vi "SVFA Power in Band.vi"   [LabVIEW 2017]
doc: "Computes the aggregate power in the <B>range</B>. The SVFA Power in Band VI operates on Power, PSD, COP, and FFT [Mag] spectra. Wire data to the <B>spectrum</B> input to determine the polymorphic instance to use or manually select the instance."
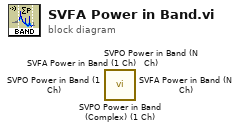
[diagram p0: block diagram]
diagram:
  n1 = call <vilib>:"SVPO Power in Band (Complex) (1 Ch).vi"() -> ()  [unwired: 19 in, 1 out]
  n2 = call <vilib>:"SVPO Power in Band (N Ch).vi"() -> ()  [unwired: 19 in, 1 out]
  n3 = call <vilib>:"SVPO Power in Band (1 Ch).vi"() -> ()  [unwired: 19 in, 1 out]
  n4 = call <vilib>:"SVFA Power in Band (N Ch).vi"() -> ()  [unwired: 17 in, 3 out]
  n5 = call <vilib>:"SVFA Power in Band (1 Ch).vi"() -> ()  [unwired: 17 in, 3 out]
